vi "VRM.Set Target.vi"(6 "Axis":T1=enum."Z", 8 "error in (no error)":errorcluster, 9 "Target Rate Limit (T/min)":dbl, 10 "Target Field (T)":dbl[](array[numeric]), 11 "Instrument.VRM in":refnum<class "Instrument.OxfordVRM.lvclass">) -> (0 "error out":errorcluster, 3 "Instrument.VRM out":refnum<class "Instrument.OxfordVRM.lvclass">)   [LabVIEW 2019, in "Instrument.OxfordVRM.lvclass"]
uses:
  Instrument.OxfordVRM.lvclass
  Typedefs/VRM Magnet Axis--Enum.ctl
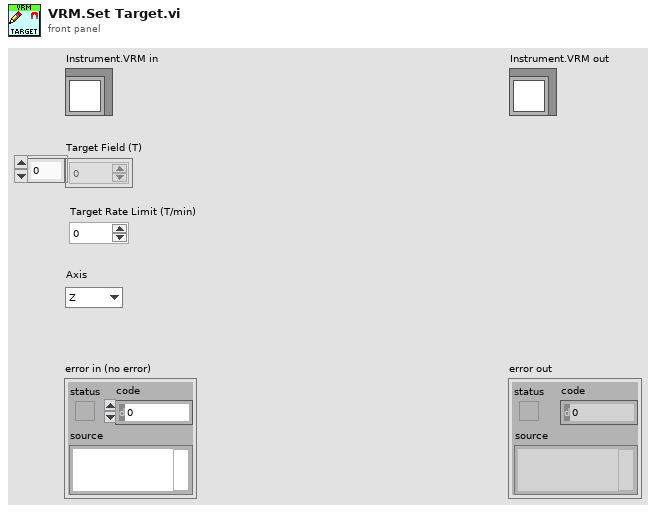
[diagram p1: front panel]
types:
  T1 = typedef "Instrument.OxfordVRM.lvclass/VRM Magnet Axis--Enum.ctl" = enum16{"X", "Y", "Z", "ALL"}
  T2 = typedef "Instrument.Cryostat.lvclass/Magnet Axis--Enum.ctl" = enum16{"X", "Y", "Z"}
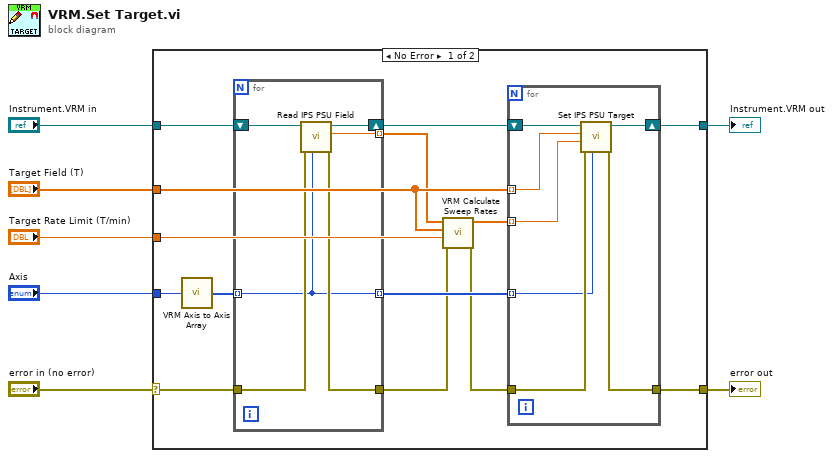
[diagram p0: block diagram]
diagram:
  n1 = case shown="No Error" "error in (no error)" {
    selector: "error in (no error)" -> [w14 w36]
    tunnel: "Target Rate Limit (T/min)" -> [w21 _]
    tunnel: [w18 w36] -> w6
    tunnel: "Target Field (T)" -> [w20 _]
    tunnel: "Instrument.VRM in" -> [w16 w35]
    tunnel: [w19 w35] -> w2
    tunnel: "Axis" -> [w17 _]
    frame No Error {
      n2 = call "VRM Axis to Axis Array.vi"("Axis"=w17) -> ("Axis Array"=w15:T2[])
      n3 = for {
        tunnel: w15 -> [w24] mode=indexing
        tunnel: w14 -> [w26]
        tunnel: [w25] -> w9
        tunnel: [w24] -> w13 mode=indexing
        tunnel: [w23] -> w12 mode=indexing
        shift-right: [w22] -> w11
        shift-left: w16 -> [w27]
        n4 = call "Read IPS PSU Field.vi"("Axis"=w24, "error in (no error)"=w26, "Instrument.OxfordVRM in"=w27) -> ("error out"=w25:errorcluster, "Power Supply Field (T)"=w23:dbl, "Instrument.OxfordVRM out"=w22:refnum<class "Instrument.OxfordVRM.lvclass">)  [unwired: 6 in]
      }
      n5 = call "VRM Calculate Sweep Rates.vi"("error in (no error)"=w9, "Sweep rate (T/min)"=w21, "Target Field (T)"=w20, "Initial Field (T)"=w12) -> ("error out"=w8:errorcluster, "Sweep Rate Field (T/min)"=w10:dbl[])  [unwired: 5 in, 1 out]
      n6 = for {
        tunnel: w13 -> [w31] mode=indexing
        shift-right: [w33] -> w19
        shift-left: w11 -> [w34]
        tunnel: w8 -> [w32]
        tunnel: [w30] -> w18
        tunnel: w20 -> [w29] mode=indexing
        tunnel: w10 -> [w28] mode=indexing
        n7 = call "Set IPS PSU Target.vi"("Axis"=w31, "error in (no error)"=w32, "Target Field Rate (T/min)"=w28, "Target Field (T)"=w29, "Instrument.OxfordVRM in"=w34) -> ("error out"=w30:errorcluster, "Instrument.OxfordVRM out"=w33:refnum<class "Instrument.OxfordVRM.lvclass">)  [unwired: 4 in, 1 out]
      }
    }
    frame Error {
    }
  }
  "Instrument.VRM out" <- w2
  "error out" <- w6
